vi "APD bias hv finder.vi"(10 "response_input":string) -> (2 "output":string)   [LabVIEW 2018]
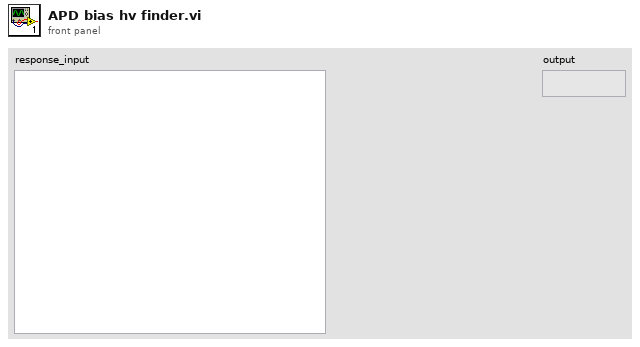
[diagram p1: front panel]
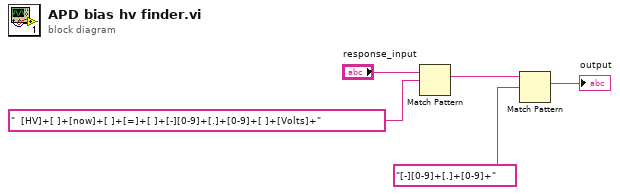
[diagram p0: block diagram]
diagram:
  n1 = Match Pattern(string="response_input", regular expression="  [HV]+[ ]+[now]+[ ]+[=]+[ ]+[-][0-9]+[.]+[0-9]+[ ]+[Volts]+") -> (match substring=w3:string)  [unwired: 1 in, 3 out]
  n2 = Match Pattern(string=w3, regular expression="[-][0-9]+[.]+[0-9]+") -> (match substring=→"output":string)  [unwired: 1 in, 3 out]
